vi "CIC_5decimate_1cycle_x410.vi"(7 "reset":bool, 8 "valid in":bool, 11 "Data in":fxp<+/-,32,14>) -> (0 "valid out":bool, 3 "Data out":fxp<+/-,32,14>)   [LabVIEW 2025]
uses:
  <vilib>/rvi/FXPMathLib/FxpConvert/subVIs/nifxpmath_Convert_SimConfig.ctl
  <vilib>/fxp/LVFixedPointQuantizationPolicyTypeDef.ctl
  <vilib>/fxp/LVFixedPointOverflowPolicyTypeDef.ctl
  <vilib>/rvi/IPIntegrationNode/IPINode_Typedef/niFpgaIPINodeSupportedFamilies.ctl
  <vilib>/rvi/FXPMathLib/FxpConvert/simVIs/DllFxpConvertTemp_sub.vi
  <vilib>/rvi/IPIntegrationNode/IPINode_Utilities/niFpgaIPINodeSimCore.vi
  <vilib>/rvi/FXPMathLib/FxpInterpret/XNode/nifxpmath_Interpret.xnode
  <vilib>/rvi/FXPMathLib/FxpMul/XNode/nifxpmath_Multiplier.xnode
  <vilib>/rvi/FXPMathLib/FxpConvert/XNode/nifxpmath_Convert.xnode
  <vilib>/rvi/XilinxIP/XIPIN_XNode/niFpgaXIPIN.xnode
  Xilinx/CIC_5decimate_1cycle_x410/xsim.dir/CIC_5decimate_1cycle_2004424183754F3994DB1309790F746C/xsimk_2004424183754F3994DB1309790F746C.dll
  <vilib>/rvi/IPIntegrationNode/IPINode_Xnode/niFpgaIPINode.xnode
  <vilib>/rvi/FXPMathLib/sim/FxpSim.dll
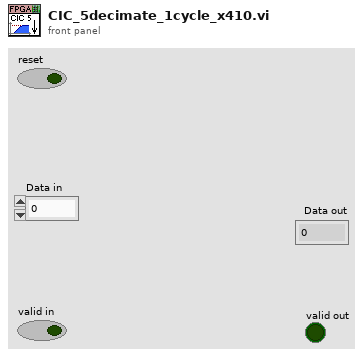
[diagram p1: front panel]
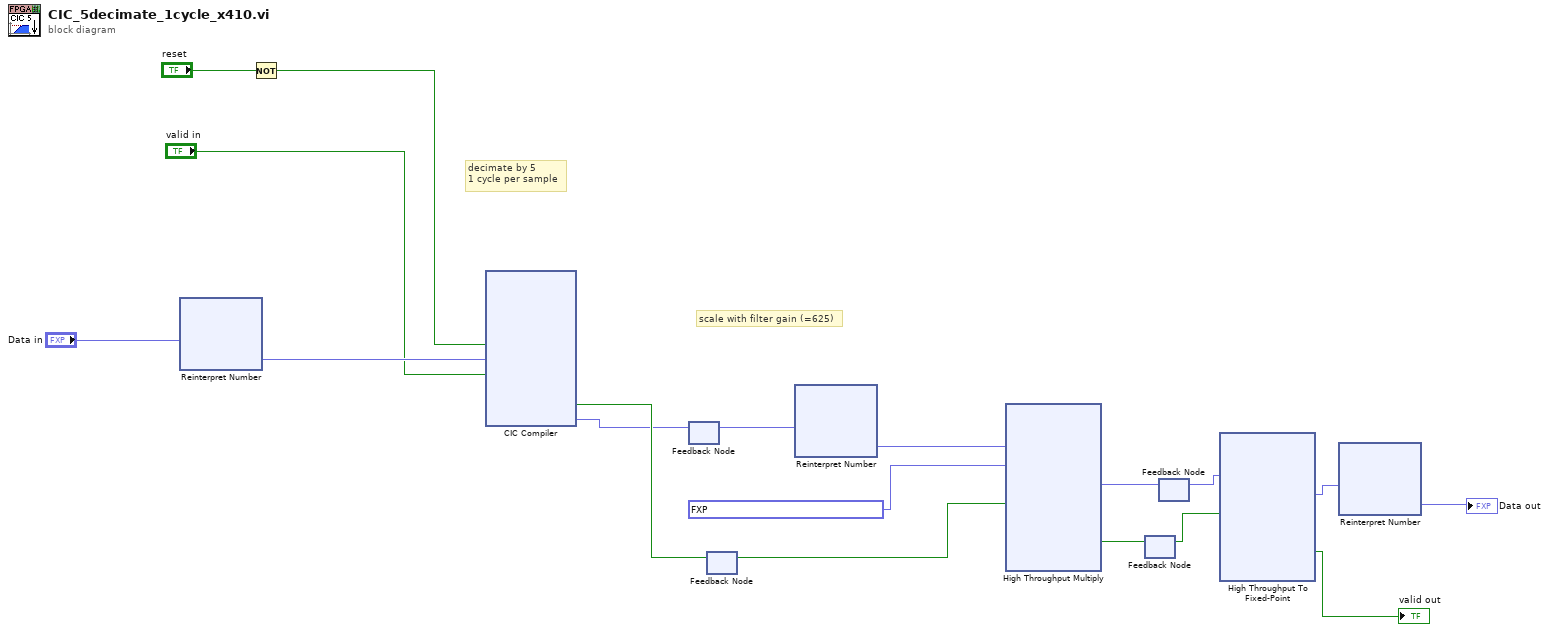
[diagram p0: block diagram]
diagram:
  # "decimate by 5\n1 cycle per sample"
  # "scale with filter gain (=625)"
  n1 = xnode "Reinterpret Number"("x"="Data in") -> ("y"=w4:fxp<+,32,32>)
  n2 = Not(x="reset") -> (.not. x?=w5:bool)
  n3 = xnode ("CIC Compiler")("aresetn"=w5, "s_axis_data_tdata"=w4, "s_axis_data_tvalid"="valid in") -> ("m_axis_data_tvalid"=w2:bool, "m_axis_data_tdata"=w1:fxp<+,48,48>)  [unwired: 1 in, 1 out]
  n4 = feedback-in #1(w1) -> ()
  n5 = feedback #1() -> (w16:fxp<+,48,48>)  [unwired: 1 in]
  n6 = feedback #2() -> (w13:bool)  [unwired: 1 in]
  n7 = feedback-in #2(w2) -> ()
  n8 = xnode "Reinterpret Number"("x"=w16) -> ("y"=w15:fxp<+/-,48,48>)
  n9 = xnode ("High Throughput Multiply")("x"=w15, "y"=fxp<+/-,32,1> 0.001600000075995922, "input valid"=w13) -> ("x*y"=w11:fxp<+/-,64,49>, "output valid"=w12:bool)  [unwired: 1 in, 1 out]
  n10 = feedback #3() -> (w8:bool)  [unwired: 1 in]
  n11 = feedback-in #3(w12) -> ()
  n12 = feedback #4() -> (w9:fxp<+/-,64,49>)  [unwired: 1 in]
  n13 = feedback-in #4(w11) -> ()
  n14 = xnode "High Throughput To Fixed-Point"("x"=w9, "input valid"=w8) -> ("y"=w7:fxp<+/-,32,32>, "output valid"=→"valid out":bool)  [unwired: 1 in, 1 out]
  n15 = xnode "Reinterpret Number"("x"=w7) -> ("y"=→"Data out":fxp<+/-,32,14>)
